vi "SDK2 multiple cameras.vi"() -> ()   [LabVIEW 2009]
panel:
  out "Shutdown":u32[](array[numeric])
  out "Initialise":u32[](array[numeric])
  out "Camera Serial numbers available":u32[](array[numeric])
  out "Camera Handles":i32[](array[numeric])
  in  "Shut Down":bool
  out "Current camera":i32
  out "Current Handle":i32
  out "totalCameras":i32
  # "This Example demonstrates how to initialise and \nshutdown multiple cameras in a single application"
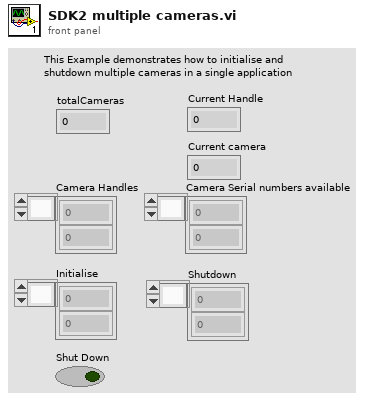
[diagram p1: front panel]
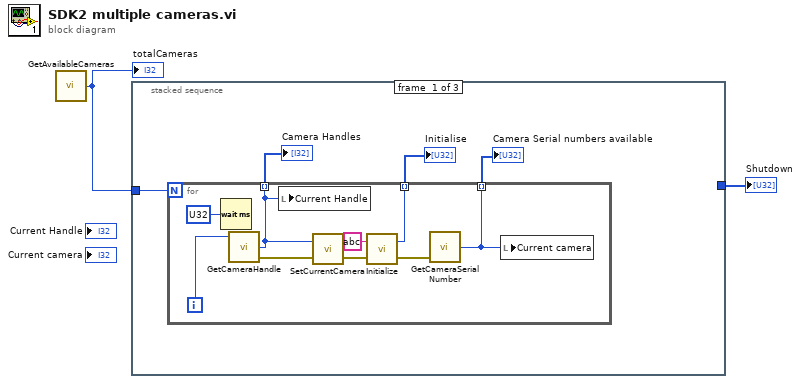
[diagram p0: block diagram]
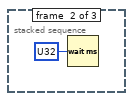
[diagram p2: hidden frame]
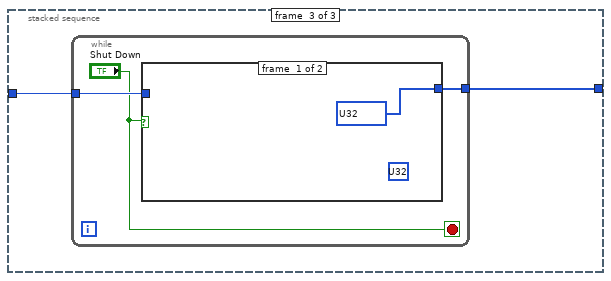
[diagram p3: hidden frame]
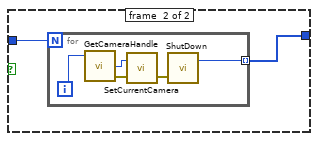
[diagram p4: hidden frame]
diagram:
  n1 = call "GetAvailableCameras.vi"() -> ("totalCameras"=w2:i32)  [unwired: 3 in, 2 out]
  "totalCameras" <- w2
  n2 = stacked-sequence {
    tunnel: w2 -> [w3 _ w17]
    tunnel: [_ _ w18] -> w1
    frame #0 {
      n3 = for {
        N: w3 -> [_]
        tunnel: [w14] -> w6 mode=indexing
        tunnel: [w8] -> w5 mode=indexing
        tunnel: [w13] -> w4 mode=indexing
        i -> [w15]
        n4 = Wait (ms)(milliseconds to wait=u32 ?) -> ()  [unwired: 1 out]
        n5 = call "GetCameraHandle.vi"("cameraIndex"=w15) -> ("error out"=w10:errorcluster, "cameraHandle"=w14:i32)  [unwired: 2 in, 1 out]
        n6 = local write "Current Handle"(w14) -> ()
        n7 = call "SetCurrentCamera.vi"("error in (no error)"=w10, "cameraHandle"=w14) -> ("error out"=w11:errorcluster)  [unwired: 1 out]
        n8 = call "Initialize.vi"("error in (no error)"=w11, "directory (\"\")"=string ? ("directory (\"\")")) -> ("error out"=w9:errorcluster, "DLL error code"=w13:u32)
        n9 = call "GetCameraSerialNumber.vi"("error in (no error)"=w9) -> ("number"=w8:i32)  [unwired: 2 in, 2 out]
        n10 = local write "Current camera"(w8) -> ()
      }
      "Camera Handles" <- w6
      "Camera Serial numbers available" <- w5
      "Initialise" <- w4
    }
    frame #1 {
      n11 = Wait (ms)(milliseconds to wait=u32 ?) -> ()  [unwired: 1 out]
    }
    frame #2 {
      n12 = while {
        tunnel: [w21] -> w18
        tunnel: w17 -> [w20]
        stop <- "Shut Down" stop-if-true
        n13 = case shown="True" "Shut Down" {
          tunnel: [u32[] ? w24] -> w21
          tunnel: w20 -> [_ w23]
          frame #0 {
            (unwired) u32 ? ("Close")
          }
          frame #1 {
            n14 = for {
              N: w23 -> [_]
              tunnel: [w29] -> w24 mode=indexing
              i -> [w27]
              n15 = call "GetCameraHandle.vi"("cameraIndex"=w27) -> ("error out"=w26:errorcluster, "cameraHandle"=w28:i32)  [unwired: 2 in, 1 out]
              n16 = call "SetCurrentCamera.vi"("error in (no error)"=w26, "cameraHandle"=w28) -> ("error out"=w25:errorcluster)  [unwired: 1 out]
              n17 = call "ShutDown.vi"("error in (no error)"=w25) -> ("DLL error code"=w29:u32)  [unwired: 1 in, 1 out]
            }
          }
        }
      }
    }
  }
  "Shutdown" <- w1
